vi "Read Matlab Params.vi"(8 "error in (no error)":errorcluster, 10 "Enum":enum16{"StartSession", "StartTrial"}(ring), 11 "TrialBasedExperiment in":refnum<class "TrialBasedExperiment.lvclass">) -> (0 "error out":errorcluster, 2 "Matlab Param Array":cluster{"Name":string, "Data":variant}[](array[cluster]), 3 "TrialBasedExperiment out":refnum<class "TrialBasedExperiment.lvclass">)   [LabVIEW 2010]
uses:
  TrialBasedExperiment.lvclass
  Matlab API/Matlab API.lvlib
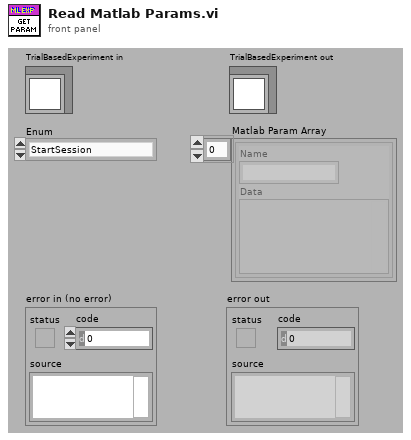
[diagram p1: front panel]
types:
  T1 = cluster{"Name":string, "Type":string, "value":string}[]
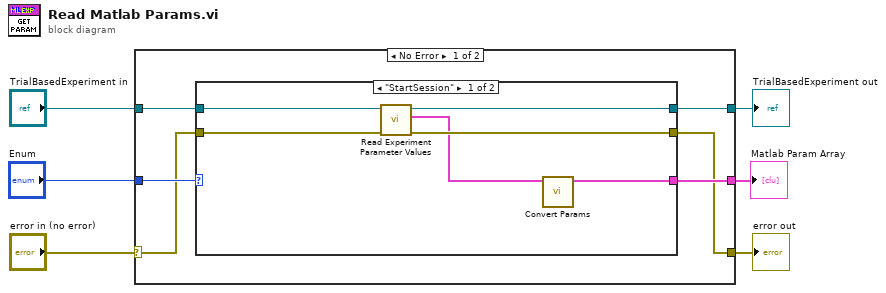
[diagram p0: block diagram]
diagram:
  n1 = case shown="No Error" "error in (no error)" {
    selector: "error in (no error)" -> [w8 w22]
    tunnel: [w7 w22] -> w5
    tunnel: [w11 w21] -> w3
    tunnel: "TrialBasedExperiment in" -> [w10 w21]
    tunnel: "Enum" -> [w12 _]
    tunnel: [w9 _] -> w1
    frame No Error {
      n2 = case shown="\"StartSession\"" w12 {
        tunnel: [w17 w20] -> w11
        tunnel: w10 -> [w18 w20]
        tunnel: [w13 _] -> w9
        tunnel: w8 -> [w16 w19]
        tunnel: [w15 w19] -> w7
        frame "StartSession" {
          n3 = call-dynamic "Read Experiment Parameter Values.vi"("error in (no error)"=w16, "TrialBasedExperiment in"=w18) -> ("error out"=w15:errorcluster, "Experiment Parameter Values"=w14:T1, "TrialBasedExperiment out"=w17:refnum<class "TrialBasedExperiment.lvclass">)  [unwired: 7 in]
          n4 = call "Convert Params.vi"("Experiment Parameter Values"=w14) -> ("Matlab Param Array"=w13:cluster{"Name":string, "Data":variant}[])  [unwired: 10 in]
        }
        frame "StartTrial", Default {
        }
      }
    }
    frame Error {
    }
  }
  "error out" <- w5
  "TrialBasedExperiment out" <- w3
  "Matlab Param Array" <- w1
